vi "Test Close.vi"(0 "Test Template in":refnum<class "niDTS Calibration Cal Execute RF Test.lvclass">, 11 "error in (no error)":errorcluster) -> (4 "Test Template out":refnum<class "niDTS Calibration Cal Execute RF Test.lvclass">, 15 "error out":errorcluster)   [LabVIEW 2015, in "niDTS Utilities.lvlib" / "niDTS Calibration Cal Execute RF Test.lvclass"]
uses:
  niDTS Calibration Cal Execute RF Test.lvclass
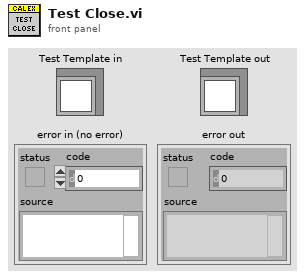
[diagram p1: front panel]
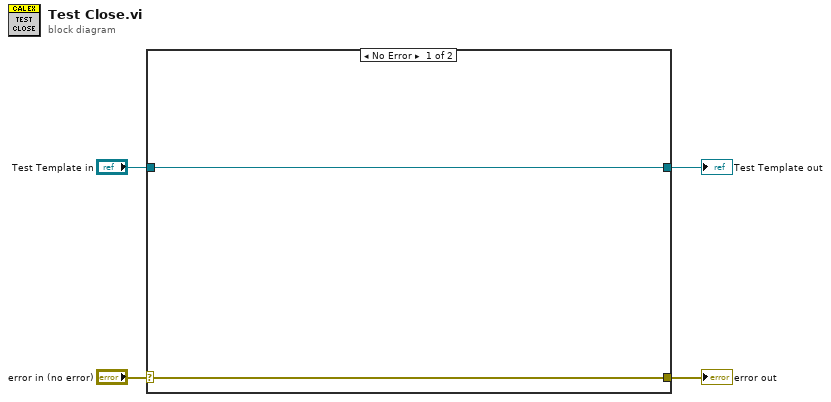
[diagram p0: block diagram]
diagram:
  n1 = case shown="No Error" "error in (no error)" {
    selector: "error in (no error)" -> [w5 w8]
    tunnel: [w5 w8] -> w3
    tunnel: "Test Template in" -> [w6 w7]
    tunnel: [w6 w7] -> w1
    frame No Error {
    }
    frame Error {
    }
  }
  "error out" <- w3
  "Test Template out" <- w1
